vi "Update Input Channel Active Status.vi"(6 "Channel Index":i32, 7 "Input Ch. Name[]":string[](array[string]), 8 "error in (no error)":errorcluster, 9 "Activate Channel?":bool, 10 "Single Channel?":bool, 11 "Plugin_UI in":refnum<class "Plugin_UI.lvclass">) -> (0 "error out":errorcluster, 2 "Error?":bool, 3 "Plugin_UI out":refnum<class "Plugin_UI.lvclass">)   [LabVIEW 2020, in "Plugin.lvlib" / "Plugin_UI.lvclass"]
doc: "Updates channel active status."
uses:
  Plugin_UI.lvclass
  C:/SVN_LabSys/labsys_lvcode/LabSys_SourceCode/builds/Libraries/LabSys Framework.lvlibp/Configurable Data Node/Configuration Interface/Configuration Interface.lvclass
  C:/SVN_LabSys/labsys_lvcode/LabSys_SourceCode/builds/Libraries/LabSys Framework.lvlibp/Process/Process/Process.lvclass
  Plugin_UI.lvclass/Plugin_UI.ctl
  Read Input Channels[].vi
  Write Input Channels[].vi
  builds/Libraries/LabSys Framework.lvlibp/Configurable Data Node/Configuration Interface/Read Module Configuration.vi
  builds/Libraries/LabSys Framework.lvlibp/Process/Process/Read Error Manager.vi
  builds/Libraries/LabSys Framework.lvlibp/Configuration Storage/Module Configuration/Read Module Name.vi
  builds/Libraries/LabSys Framework.lvlibp/Configuration Storage/Module Configuration/Module Configuration.lvclass
  Channels/Input Channels/Input Channels.lvclass
  builds/Libraries/LabSys Framework.lvlibp/Error Manager/Error Manager/Error Manager.lvclass
  builds/Libraries/Shared GUI Library.lvlibp
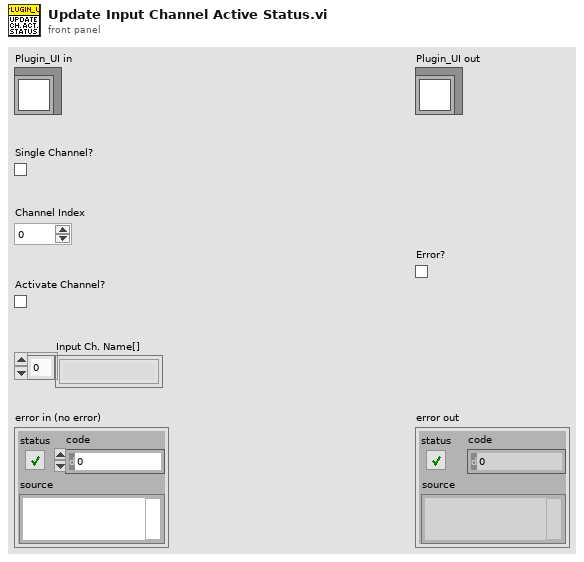
[diagram p1: front panel]
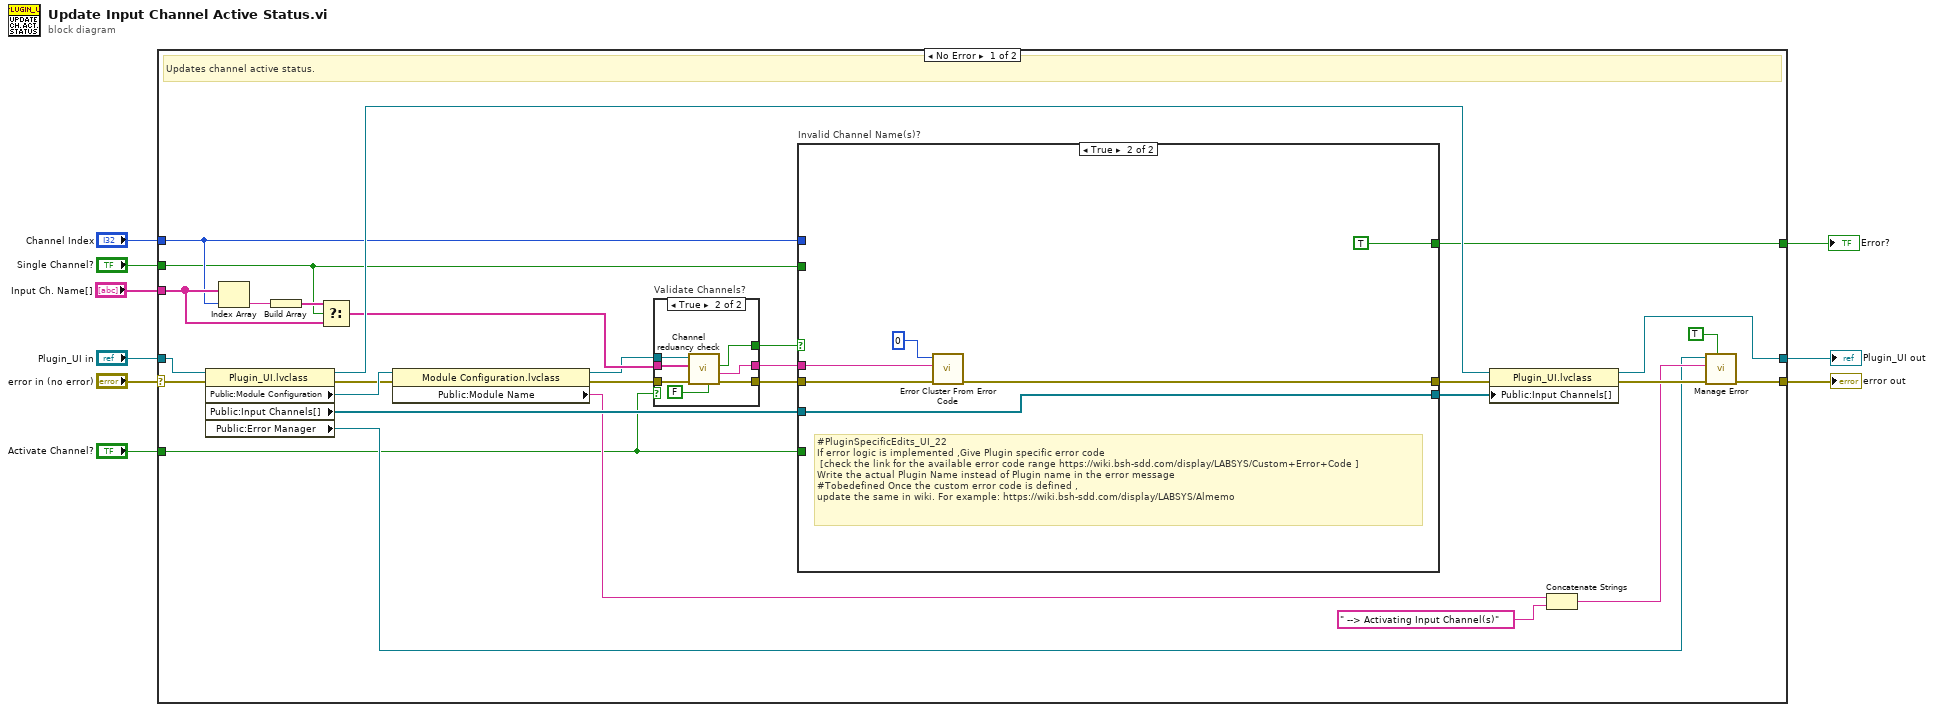
[diagram p0: block diagram]
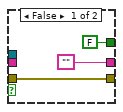
[diagram p2: hidden frame]
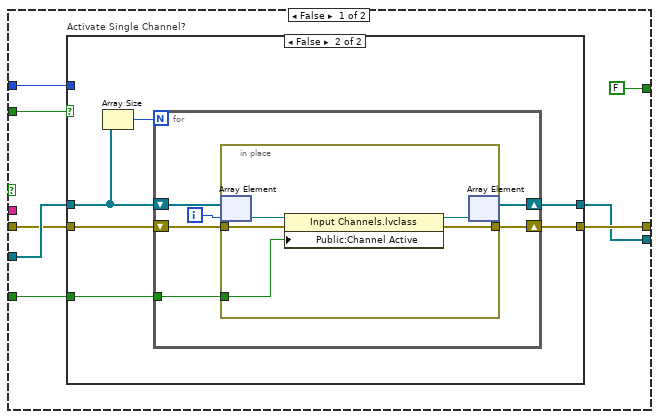
[diagram p3: hidden frame]
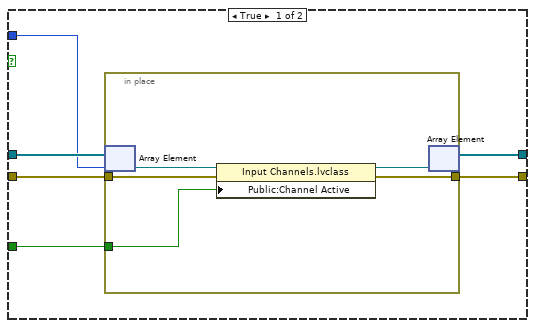
[diagram p4: hidden frame]
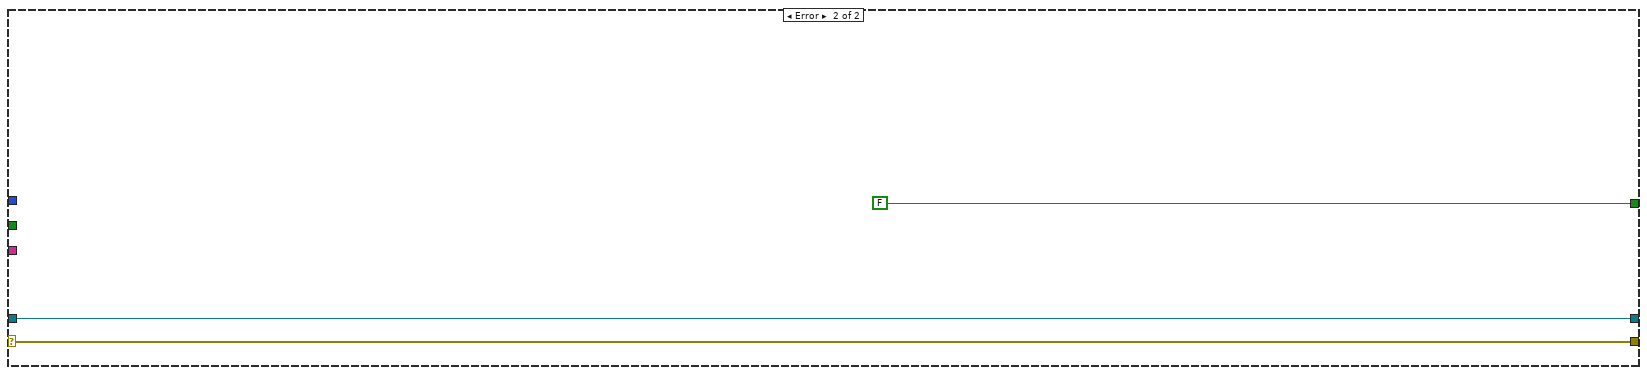
[diagram p5: hidden frame]
diagram:
  n1 = case shown="No Error" "error in (no error)" {
    selector: "error in (no error)" -> [w37 w93]
    tunnel: "Plugin_UI in" -> [w38 w92]
    tunnel: [w21 w93] -> w7
    tunnel: "Channel Index" -> [w27 _]
    tunnel: "Activate Channel?" -> [w10 _]
    tunnel: [w32 w92] -> w4
    tunnel: "Single Channel?" -> [w24 _]
    tunnel: "Input Ch. Name[]" -> [w28 _]
    tunnel: [w11 FALSE ("Error?")] -> w1
    frame No Error {
      # "Updates channel active status."
      n2 = property class="Plugin_UI.lvclass"(reference=w38, error in=w37) -> (reference out=w33:refnum<class "Plugin_UI.lvclass">, error out=w18:errorcluster, "Public:Module Configuration"=w19:refnum<class "Module Configuration.lvclass">, "Public:Input Channels[]"=w36:refnum<class "Input Channels.lvclass">[], "Public:Error Manager"=w12:refnum<data-value>)
      n3 = Index Array(array=w28, index=w27) -> (element=w26:string)
      n4 = Build Array(w26) -> (w25:string[])
      n5 = Select(t=w25, s=w24, f=w28) -> (s? t:f=w29:string[])
      n6 = property class="Module Configuration.lvclass"(reference=w19, error in=w18) -> (reference out=w16:refnum<class "Module Configuration.lvclass">, error out=w17:errorcluster, "Public:Module Name"=w13:string)
      n7 = case "Validate Channels?" shown="True" w10 {
        tunnel: [w41 w48] -> w30
        tunnel: w29 -> [_ w47]
        tunnel: [FALSE ("Channel Configuration Found(F)") w46] -> w23
        tunnel: ["" w45] -> w20
        tunnel: w17 -> [w41 w44]
        tunnel: w16 -> [_ w43]
        frame False {
        }
        frame True {
          n8 = call "Channel reduancy check.vi"("Show Pop up"=FALSE, "error in"=w44, "New Channel Name[]"=w47, "Module configuration in"=w43) -> ("error out"=w48:errorcluster, "Error message"=w45:string, "Channel Configuration Found(F)"=w46:bool)  [unwired: 4 in, 1 out]
        }
      }
      n9 = case "Invalid Channel Name(s)?" shown="True" w23 {
        tunnel: w36 -> [w56 w90]
        tunnel: w10 -> [w55 _]
        tunnel: [w54 w87] -> w35
        tunnel: [w53 w90] -> w34
        tunnel: w30 -> [w52 w88]
        tunnel: w27 -> [w51 _]
        tunnel: w24 -> [w50 _]
        tunnel: w20 -> [_ w86]
        tunnel: [FALSE ("Error?") TRUE ("Error?")] -> w11
        frame False {
          n10 = case "Activate Single Channel?" shown="False" w50 {
            tunnel: w56 -> [w62 w69]
            tunnel: w55 -> [w61 w73]
            tunnel: [w60 w72] -> w54
            tunnel: [w59 w71] -> w53
            tunnel: w52 -> [w58 w70]
            tunnel: w51 -> [w57 _]
            frame True {
              n11 = in-place {
                in-place-border: w58 -> [w65]
                in-place-border: w61 -> [w63]
                in-place-border: [w66] -> w60
                n12 = in-place-array #1(w62, w57) -> (w64:refnum<class "Input Channels.lvclass">)
                n13 = property class="Input Channels.lvclass"(reference=w64, error in=w65, "Public:Channel Active"=w63) -> (reference out=w67:refnum<class "Input Channels.lvclass">, error out=w66:errorcluster)
                n14 = in-place-array #1(w67) -> (w59:refnum<class "Input Channels.lvclass">[])  [unwired: 1 out]
              }
            }
            frame False {
              n15 = Array Size(array=w69) -> (size(s)=w68:i32)
              n16 = for {
                N: w68 -> [_]
                tunnel: w73 -> [w78]
                shift-right: [w77] -> w72
                shift-left: w70 -> [w75]
                shift-right: [w76] -> w71
                shift-left: w69 -> [w79]
                i -> [w74]
                n17 = in-place {
                  in-place-border: w75 -> [w82]
                  in-place-border: w78 -> [w80]
                  in-place-border: [w83] -> w77
                  n18 = in-place-array #2(w79, w74) -> (w81:refnum<class "Input Channels.lvclass">)
                  n19 = property class="Input Channels.lvclass"(reference=w81, error in=w82, "Public:Channel Active"=w80) -> (reference out=w84:refnum<class "Input Channels.lvclass">, error out=w83:errorcluster)
                  n20 = in-place-array #2(w84) -> (w76:refnum<class "Input Channels.lvclass">[])  [unwired: 1 out]
                }
              }
            }
          }
        }
        frame True {
          # "#PluginSpecificEdits_UI_22\nIf error logic is implemented ,Give Plugin specific error code\n [check the link for the available error code range https://wiki.bsh-sdd.com/display/LABSYS/Custom+Error+Code ]\nWrite the actual Plugin Name instead of Plugin name in the error message\n#Tobedefined Once the custom error code is defined , \nupdate the same in wiki. For example: https://wiki.bsh-sdd.com/display/LABSYS/Almemo"
          n21 = call <vilib>:"Error Cluster From Error Code.vi"("error in (no error)"=w88, "error message (\"\")"=w86, "error code (0)"=0) -> ("error out"=w87:errorcluster)  [unwired: 6 in]
        }
      }
      n22 = property class="Plugin_UI.lvclass"(reference=w33, error in=w35, "Public:Input Channels[]"=w34) -> (reference out=w32:refnum<class "Plugin_UI.lvclass">, error out=w22:errorcluster)
      n23 = Concatenate Strings(w13, " --> Activating Input Channel(s)" ("Error Location")) -> (w14:string)
      n24 = call "Manage Error.vi"("Clear Errors (F)"=TRUE, "error in (no error)"=w22, "Error Location"=w14, "Error Manager in"=w12) -> ("error out"=w21:errorcluster)  [unwired: 6 in, 1 out]
    }
    frame Error {
    }
  }
  "error out" <- w7
  "Plugin_UI out" <- w4
  "Error?" <- w1
